vi "Main.vi"() -> ()   [LabVIEW 2024]
uses:
  <vilib>/Utility/file.llb/Read Delimited Spreadsheet (string).vi
panel:
  out "Categories":string[](array[string])
  out "all rows":string[][](array[string])
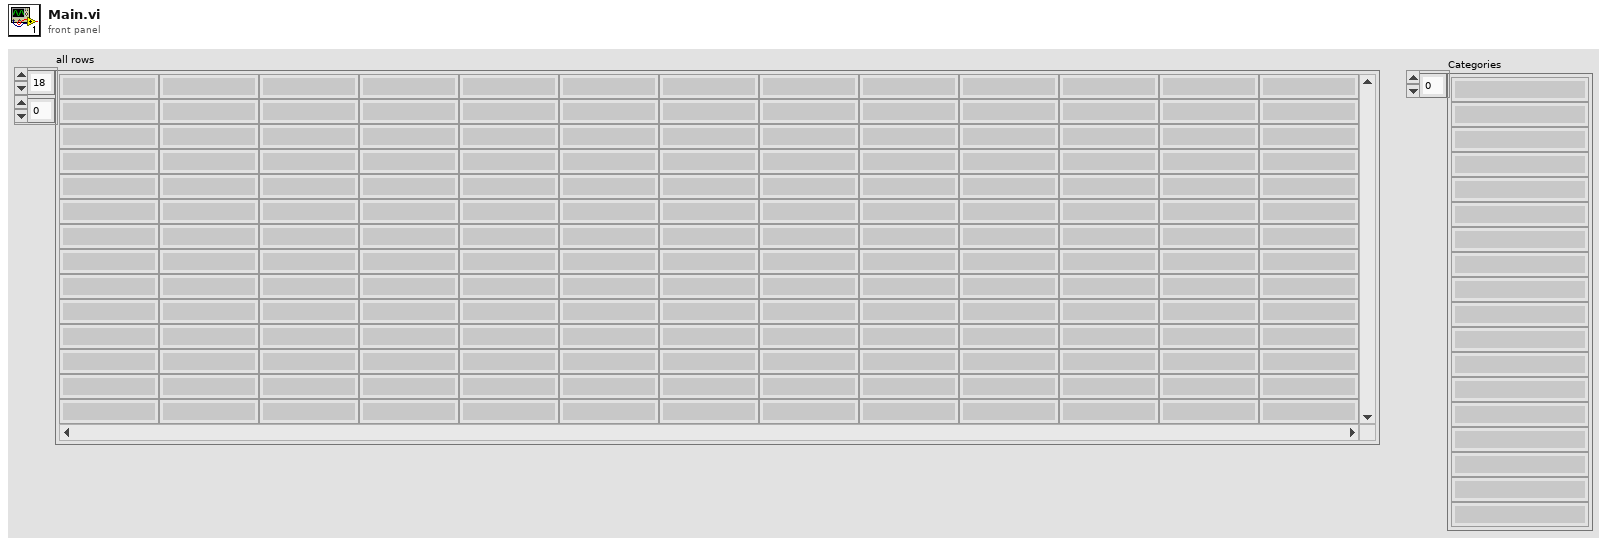
[diagram p1: front panel]
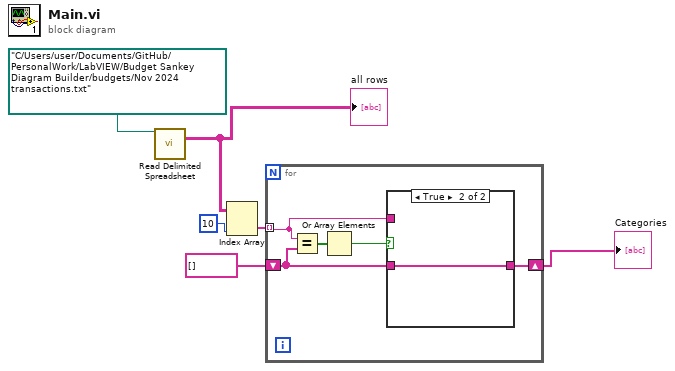
[diagram p0: block diagram]
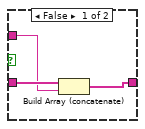
[diagram p2: hidden frame]
diagram:
  n1 = call-poly <vilib>:"Read Delimited Spreadsheet.vi"("file path (dialog if empty)"=path "C:/Users/user/Documents/GitHub/PersonalWork/LabVIEW/Budget Sankey Diagram Builder/budgets/Nov 2024 transactions.txt") -> ("all rows"=w6:string[][])  [unwired: 9 in, 5 out]
  "all rows" <- w6
  n2 = Index Array(array=w6, index (col)=10 ("index")) -> (element=w4:string[])  [unwired: 1 in]
  n3 = for {
    shift-right: [w8] -> w3
    shift-left: string[] [] -> [w9]
    tunnel: w4 -> [w7] mode=indexing
    n4 = Equal?(x=w7, y=w9) -> (x = y?=w11:bool[])
    n5 = Or Array Elements(Boolean array=w11) -> (logical OR=w10:bool)
    n6 = case shown="True" w10 {
      tunnel: w9 -> [w14 w15]
      tunnel: [w13 w15] -> w8
      tunnel: w7 -> [w12 _]
      frame False {
        n7 = Build Array (concatenate)(w14, w12) -> (w13:string[])
      }
      frame True {
      }
    }
  }
  "Categories" <- w3
